vi "fgv - reset.vi"(8 "error in (no error)":errorcluster, 10 "Write Data (F)":bool, 11 "Operation":enum16{"Read", "Write"}(ring)) -> (0 "error out":errorcluster, 2 "Read Data":bool)   [LabVIEW 2016]
panel:
  # "fgv - reset"
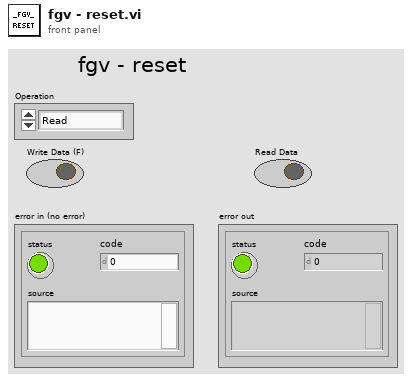
[diagram p1: front panel]
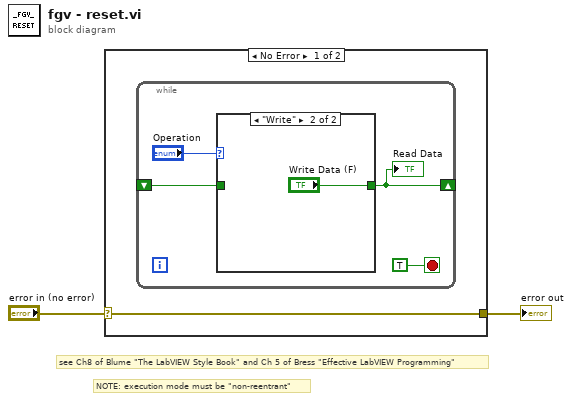
[diagram p0: block diagram]
diagram:
  # "NOTE: execution mode must be \"non-reentrant\""
  # "see Ch8 of Blume \"The LabVIEW Style Book\" and Ch 5 of Bress \"Effective LabVIEW Programming\""
  n1 = case shown="No Error" "error in (no error)" {
    selector: "error in (no error)" -> [w3 w10]
    tunnel: [w3 w10] -> w1
    frame No Error {
      n2 = while {
        shift-right: [w4] -> _
        shift-left: _ -> [w6]
        stop <- TRUE stop-if-true
        n3 = case shown="\"Write\"" "Operation" {
          tunnel: [w8 "Write Data (F)"] -> w4
          tunnel: w6 -> [w8 _]
          frame "Read", Default {
          }
          frame "Write" {
          }
        }
        "Read Data" <- w4
      }
    }
    frame Error {
    }
  }
  "error out" <- w1
